vi "change_array32.vi"(3 "IN":u32[](array[numeric]) format="%x") -> (1 "change":bool)   [LabVIEW 2019, in "Logik.lvlib"]
uses:
  Logik.lvlib
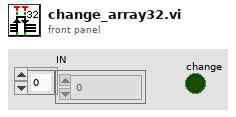
[diagram p1: front panel]
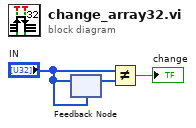
[diagram p0: block diagram]
diagram:
  n1 = feedback #1("IN") -> (w3:u32[])
  n2 = feedback-in #1("IN") -> ()
  n3 = Not Equal?(x="IN", y=w3) -> (x != y?=→"change":bool)
